vi "2D Array Sorter.vi"(9 "Sorting Index":i32, 10 "Array":string[][](array[string])=[["Horse", "1", "2"], ["Monkey", "100", "200"], ["elephant", "1000", "2000"], ["chicken", "10000", "20000"]]) -> (3 "sorted array":string[][](array[string]))   [LabVIEW 2021]
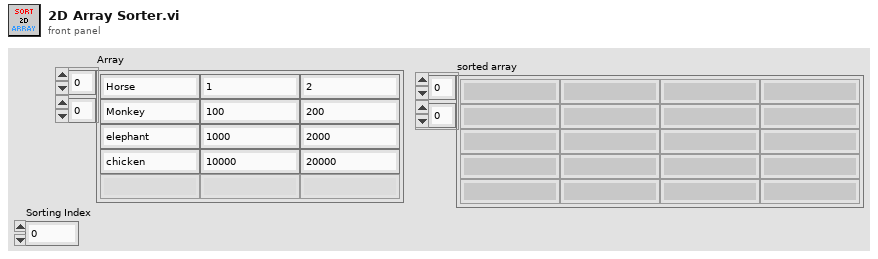
[diagram p1: front panel]
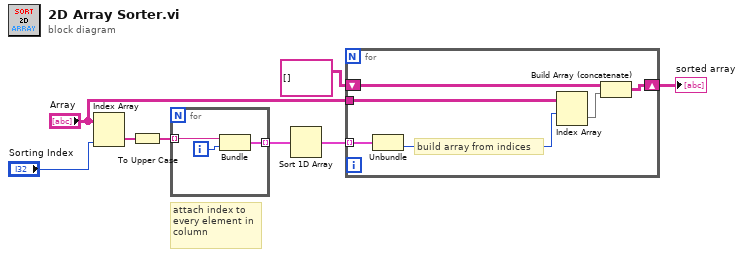
[diagram p0: block diagram]
diagram:
  # "attach index to \nevery element in\ncolumn"
  n1 = Index Array(array="Array", index (col)="Sorting Index") -> (element=w4:string[])  [unwired: 1 in]
  n2 = To Upper Case(1:w4) -> (0:w3:string[])
  n3 = for {
    tunnel: w3 -> [w11] mode=indexing
    tunnel: [w9] -> w8 mode=indexing
    i -> [w10]
    n4 = Bundle("String"=w11, w10) -> (w9:cluster{"String":string, i32})  [unwired: 1 in]
  }
  n5 = Sort 1D Array(array=w8) -> (sorted array=w5:cluster{"String":string, i32}[])
  n6 = for {
    tunnel: "Array" -> [w15]
    shift-right: [w13] -> w2
    shift-left: string[][] [] ("Array") -> [w14]
    tunnel: w5 -> [w17] mode=indexing
    # "build array from indices"
    n7 = Unbundle(w17) -> (w16:i32)  [unwired: 1 out]
    n8 = Index Array(array=w15, index (row)=w16) -> (element=w12:string[])  [unwired: 1 in]
    n9 = Build Array (concatenate)(w14, w12) -> (w13:string[][])
  }
  "sorted array" <- w2
